vi "2 HeadingChooser.vi"(11 "CurrentMission":refnum<class "GenericMission.lvclass">) -> (2 "Optimal Heading Out":dbl, 3 "Goodness Functions":T3)   [LabVIEW 2011]
doc: "The Heading Chooser VI is responsible for finding the optimal heading for the boat in order to reach the waypoint. It uses fuzzy-logic inspired goodness function logic to choose a heading. Specifically, the VI takes 3 goodness function curves and makes a weighted combination of them, choosing the heading with the highest total goodness.\n\nThis VI does not contain any code that would limit the component goodness functions to just 3 or to the specific ones of 'target', 'no sail', and 'change'. Only the labels would need changing."
uses:
  2 Globals/2 Global.vi
  2 Globals/2 TuningConstants.vi
  2 Typedefs/Goodness Weightings.ctl
  2 Typedefs/Goodness Fns Indicator.ctl
  2 Typedefs/tacking attempt.ctl
  2 Classes/Missions/GenericMission/GenericMission.lvclass
panel:
  out "Tacking Attempt":T1
  out "tack start time":timestamp
  out "Goodness Weightings":T2={"Target Importance"=0.98, "No Sail Importance"=1.0, "Change Importance"=0.2, "Pure Waypoint \nImportance"=0.0, "Pure Wind \nImportance"=0.0} {"Pure Wind \nImportance" min=0.0 step=0.2; "Pure Waypoint \nImportance" min=0.0 step=0.2; "Change Importance" min=0.0 step=0.2; "No Sail Importance" min=0.0 step=0.2; "Target Importance" min=0.0 step=0.2}
  out "Latest Optimal Heading":dbl
  # "huh???\nTODO: talk to NI about this"
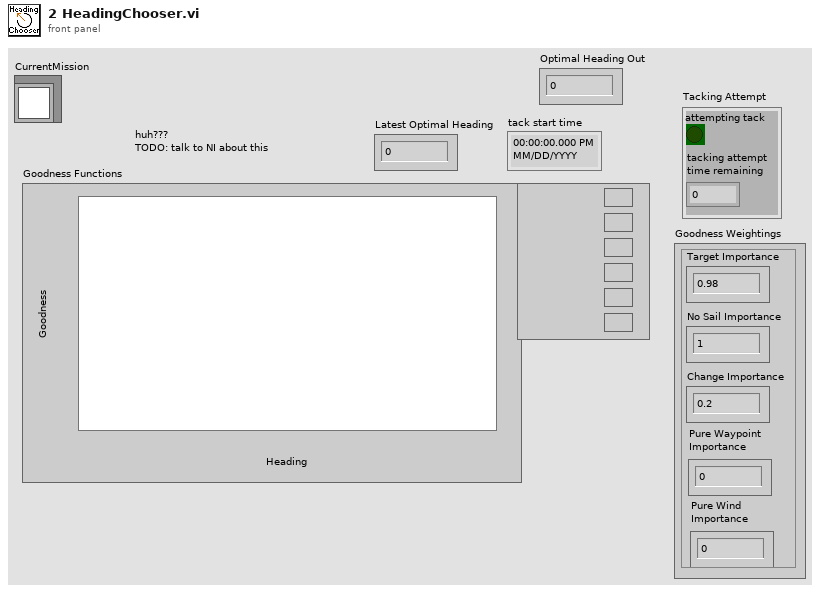
[diagram p1: front panel]
types:
  T1 = typedef "tacking attempt.ctl" = cluster{"attempting tack":bool, "tacking attempt\ntime remaining":dbl}
  T2 = typedef "Goodness Weightings.ctl" = cluster{"Target Importance":dbl, "No Sail Importance":dbl, "Change Importance":dbl, "Pure Waypoint \nImportance":dbl, "Pure Wind \nImportance":dbl}
  T3 = typedef "Goodness Fns Indicator.ctl" = cluster{dbl, dbl, dbl[][]}
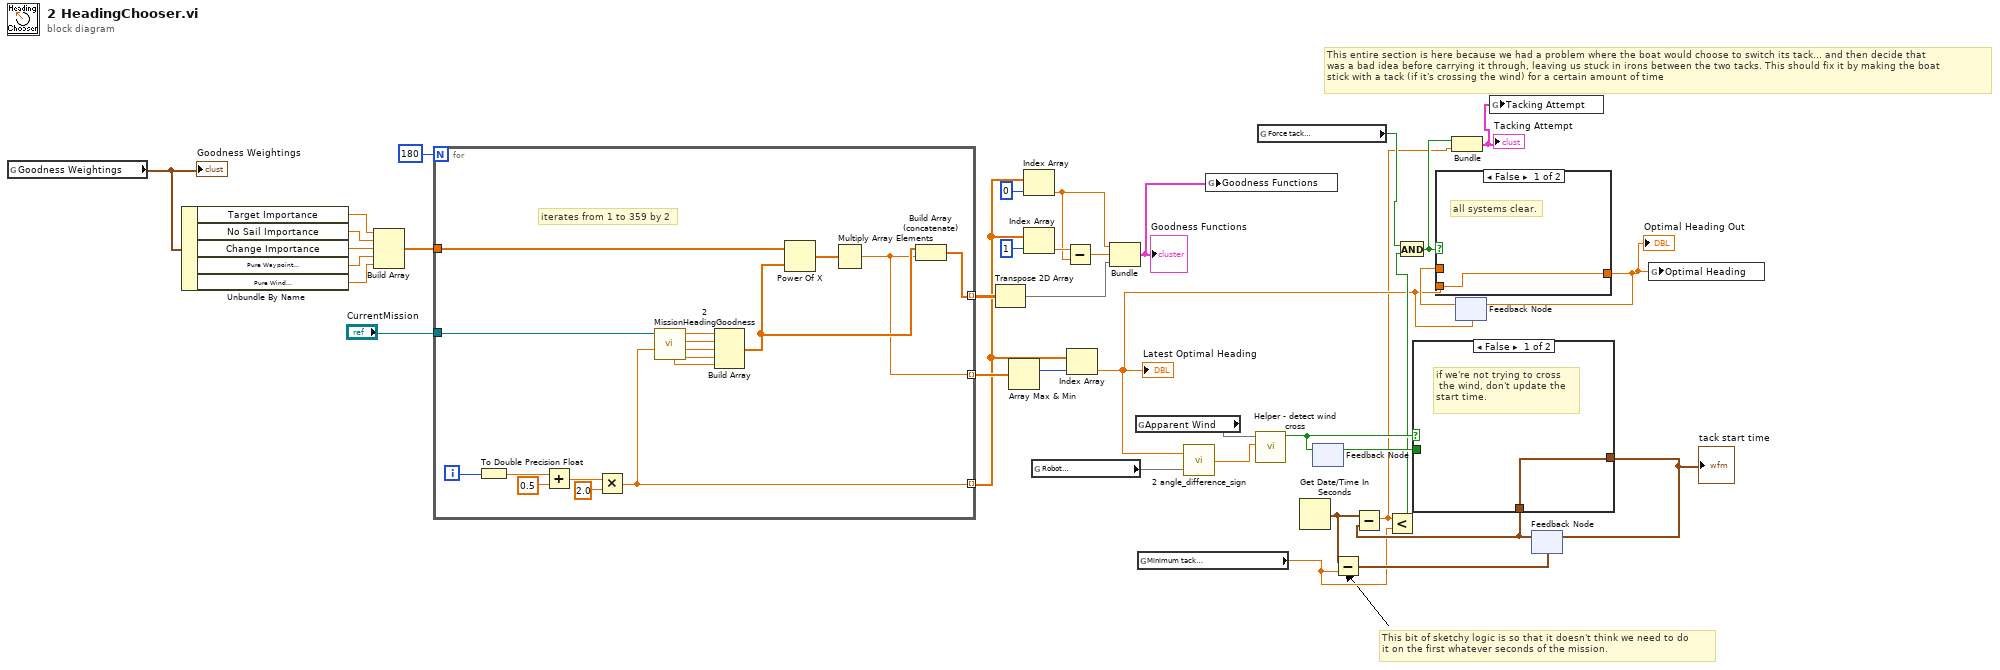
[diagram p0: block diagram]
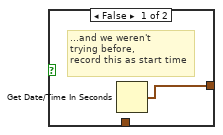
[diagram p4: hidden frame]
diagram:
  # "This entire section is here because we had a problem where the boat would choose to switch its tack... and then decide that\nwas a bad idea before carrying it through, leaving us stuck in irons between the two tacks. This should fix it by making the boat\nstick with a tack (if it's crossing the wind) for a certain amount of time"
  # "This bit of sketchy logic is so that it doesn't think we need to do\nit on the first whatever seconds of the mission."
  n1 = global read "2 TuningConstants.vi" "Goodness Weightings"() -> (w8:T2)
  "Goodness Weightings" <- w8
  n2 = Unbundle By Name(w8) -> ("Target Importance"=w5:dbl, "No Sail Importance"=w6:dbl, "Change Importance"=w7:dbl, "Pure Waypoint \nImportance"=w4:dbl, "Pure Wind \nImportance"=w3:dbl)
  n3 = Build Array(w5, w6, w7, w4, w3) -> (w2:dbl[])
  n4 = for {
    N: 180 -> [_]
    tunnel: [w47] -> w31 mode=indexing
    tunnel: "CurrentMission" -> [w39]
    tunnel: [w54] -> w32 mode=indexing
    tunnel: [w40] -> w27 mode=indexing
    tunnel: w2 -> [w46]
    i -> [w55]
    # "iterates from 1 to 359 by 2"
    n5 = To Double Precision Float(number=w55) -> (double precision float=w52:dbl)
    n6 = Add(x=w52, y=0.5) -> (x+y=w51:dbl)
    n7 = Multiply(x=w51, y=2.0) -> (x*y=w40:dbl)
    n8 = call "2 MissionHeadingGoodness.vi"("Heading to Test"=w40, "CurrentMission"=w39) -> ("Pure Waypoint Goodness"=w42:dbl, "Direction Change Goodness"=w43:dbl, "No-Sail Goodness"=w44:dbl, "Target Goodness"=w45:dbl, "Pure Wind Goodness"=w41:dbl)  [unwired: 5 in]
    n9 = Build Array(w45, w44, w43, w42, w41) -> (w49:dbl[])
    n10 = Power Of X(1:w49, 2:w46) -> (0:w48:dbl[])
    n11 = Multiply Array Elements(1:w48) -> (0:w47:dbl)
    n12 = Build Array (concatenate)(w49, w47) -> (w54:dbl[])
  }
  n13 = Transpose 2D Array(2D array=w32) -> (transposed array=w28:dbl[][])
  n14 = Array Max & Min(array=w31) -> (max index (indices)=w34:i32)  [unwired: 3 out]
  n15 = Index Array(array=w27, index=0) -> (element=w30:dbl)
  n16 = Index Array(array=w27, index=1) -> (element=w37:dbl)
  n17 = global read "2 Global.vi" "Robot\nHeading"() -> (w25)
  n18 = Subtract(x=w37, y=w30) -> (x-y=w29:dbl)
  n19 = Index Array(array=w27, index=w34) -> (element=w14:dbl)
  "Latest Optimal Heading" <- w14
  n20 = Bundle(w30, w29, w28) -> (w33:cluster{dbl, dbl, dbl[][]})  [unwired: 1 in]
  "Goodness Functions" <- w33
  n21 = global read "2 Global.vi" "Apparent Wind"() -> (w26)
  n22 = global read "2 TuningConstants.vi" "Minimum tack\ntry time?"() -> (w13:dbl)
  n23 = call "2 angle_difference_sign.vi"("Angle 2"=w25, "Angle 1"=w14) -> ("Difference"=w24:dbl)
  n24 = global write "2 Global.vi" "Goodness Functions"(w33) -> ()
  n25 = call "Helper - detect wind cross.vi"("Heading Change"=w24, "Apparent Wind"=w26) -> ("Crossing Wind?"=w23:bool)  [unwired: 9 in]
  n26 = global read "2 TuningConstants.vi" "Force tack\nattempt?"() -> (w12:bool)
  n27 = Get Date/Time In Seconds() -> (seconds since 1Jan1904=w19:timestamp)
  n28 = feedback #1() -> (w22:bool)  [unwired: 1 in]
  n29 = feedback-in #1(w23) -> ()
  n30 = Subtract(x=w19, y=w13) -> (x-y=w18:timestamp)
  n31 = feedback #2(w14) -> (w15:dbl)
  n32 = feedback #3(w18) -> (w20:timestamp)
  n33 = Subtract(x=w19, y=w20) -> (x-y=w10:dbl)
  n34 = Less?(x=w10, y=w13) -> (x < y?=w17:bool)
  n35 = And(x=w12, y=w17) -> (x .and. y?=w11:bool)
  n36 = case shown="False" w23 {
    tunnel: w22 -> [_ w59]
    tunnel: [w56 w58] -> w21
    tunnel: w20 -> [w56 w57]
    frame False {
      # "if we're not trying to cross\n the wind, don't update the\nstart time."
    }
    frame True {
      # "if we're trying to cross the wind..."
      n37 = case shown="True" w59 {
        tunnel: [w60 w61] -> w58
        tunnel: w57 -> [_ w61]
        frame False {
          # "...and we weren't\ntrying before,\nrecord this as start time"
          n38 = Get Date/Time In Seconds() -> (seconds since 1Jan1904=w60:timestamp)
        }
        frame True {
          # "and we were trying to\nbefore, keep counting"
        }
      }
    }
  }
  "tack start time" <- w21
  n39 = case shown="False" w11 {
    tunnel: w14 -> [w62 _]
    tunnel: [w62 w63] -> w16
    tunnel: w15 -> [_ w63]
    frame False {
      # "all systems clear."
    }
    frame True {
      # "if it's been less than 5\nseconds since we started\ntrying to cross the wind,\ndon't let the boat change its\nmind"
    }
  }
  "Optimal Heading Out" <- w16
  n40 = Bundle(w11, w10) -> (w9:cluster{bool, dbl})  [unwired: 1 in]
  "Tacking Attempt" <- w9
  n41 = feedback-in #2(w16) -> ()
  n42 = global write "2 Global.vi" "Tacking Attempt"(w9) -> ()
  n43 = feedback-in #3(w21) -> ()
  n44 = global write "2 Global.vi" "Optimal Heading"(w16) -> ()
